vi "arduino_serial.vi"() -> ()   [LabVIEW 2018]
uses:
  <vilib>/Instr/_visa.llb/VISA Configure Serial Port (Instr).vi
panel:
  out "resulting string":string
  out "error out 2":errorcluster
  in  "milliseconds to wait":u32
  out "error out":errorcluster
  in  "VISA resource name":refnum<visa-resource-name>
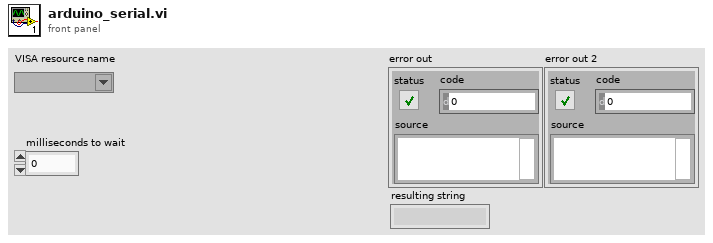
[diagram p1: front panel]
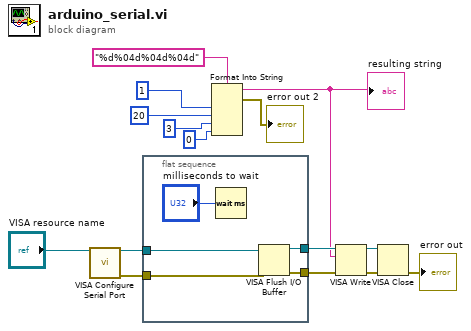
[diagram p0: block diagram]
diagram:
  n1 = call-poly "VISA Configure Serial Port"("VISA resource name"="VISA resource name") -> ("VISA resource name out"=w9:refnum<visa-resource-name>, "error out"=w8:errorcluster)  [unwired: 13 in]
  n2 = flat-sequence {
    tunnel: [w20] -> w14
    tunnel: [w19] -> w13
    tunnel: w9 -> [w17]
    tunnel: w8 -> [w16]
    frame #0 {
      n3 = Wait (ms)(milliseconds to wait="milliseconds to wait") -> ()  [unwired: 1 out]
      n4 = VISA Flush I/O Buffer(VISA resource name=w17, error in (no error)=w16) -> (VISA resource name out=w20:refnum<visa-resource-name>, error out=w19:errorcluster)  [unwired: 1 in]
    }
  }
  n5 = Format Into String(format string="%d%04d%04d%04d", 1 ("input 1"), 20 ("input 2"), 3 ("input 3"), 0 ("input 4")) -> (resulting string=w4:string, error out=→"error out 2":errorcluster)  [unwired: 2 in]
  "resulting string" <- w4
  n6 = VISA Write(VISA resource name=w14, write buffer=w4, error in (no error)=w13) -> (VISA resource name out=w12:refnum<visa-resource-name>, error out=w11:errorcluster)  [unwired: 1 out]
  n7 = VISA Close(VISA resource name=w12, error in (no error)=w11) -> (error out=→"error out":errorcluster)
